vi "DataLog Create Tag Log Directory.vi"(0 "tag log directory":path, 1 "no initial? (false)":bool, 5 "initial number (NaN)":dbl=nan format="%.2f", 7 "initial tag config":T1 {"logging parameters" format="%.2e"; "precision" items=["0", "1", "2", "3", "4", "5", "6", "7", "8", "9", "10", "11", "12", "13", "14", "15", "16", "17"]; "limit delay" format="%.2e"; "deadband" format="%.2e"}, 9 "initial string (\"\")":string, 11 "error in (no error)":errorcluster) -> (4 "dup tag log directory":path, 15 "error out":errorcluster)   [LabVIEW 2012]
doc: "Create a new tag log directory if no such directory exists yet. On creation, a single point with the current time and specified initial value is logged in case of a number tag. In case of a string tag, an undefined string value is logged."
uses:
  typedefs/clusters/t_DataLog Tag Config.ctl
  typedefs/t_DataLog Temporal Types.ctl
  typedefs/t_DataLog Value Types.ctl
  typedefs/t_DataLog Numerical Format.ctl
  typedefs/t_DataLog Logging Algorithms.ctl
  typedefs/clusters/t_DataLog Point.ctl
  glb_DataLog MCVD.vi
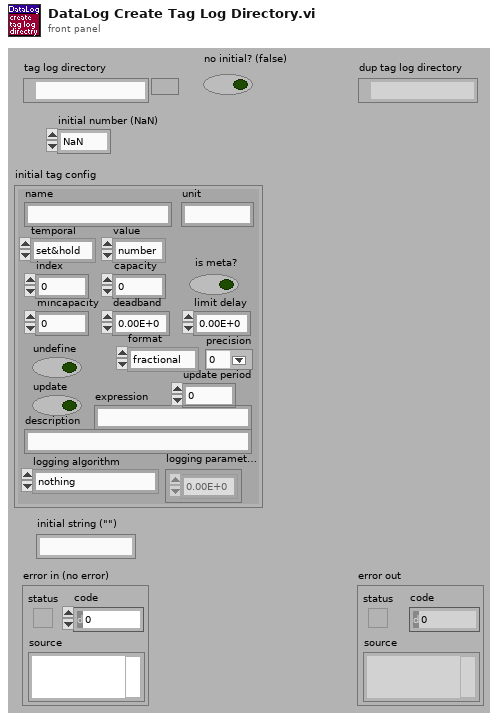
[diagram p1: front panel]
types:
  T1 = typedef "t_DataLog Tag Config.ctl" = cluster{"name":string, "unit":string, "temporal":T2, "value":T3, "index":i32, "capacity":i32, "is meta?":bool, "mincapacity":i32, "deadband":dbl, "limit delay":dbl, "format":T4, "precision":u8, "undefine":bool, "update":bool, "update period":u16, "expression":string, "description":string, "logging algorithm":T5, "logging parameters":dbl[]}
  T2 = typedef "t_DataLog Temporal Types.ctl" = enum16{"set&hold", "sample", "event"}
  T3 = typedef "t_DataLog Value Types.ctl" = enum16{"number", "string"}
  T4 = typedef "t_DataLog Numerical Format.ctl" = enum8{"fractional", "exponential", "engineering"}
  T5 = typedef "t_DataLog Logging Algorithms.ctl" = enum16{"nothing", "changes", "everything", "every Nth", "time threshold", "value threshold + prior", "t or v threshold", "t or v threshold + prior"}
  T6 = enum16{"deny read/write", "deny write-only", "deny none"}
  T7 = typedef "t_DataLog Point.ctl" = cluster{"time":dbl, "value":dbl}
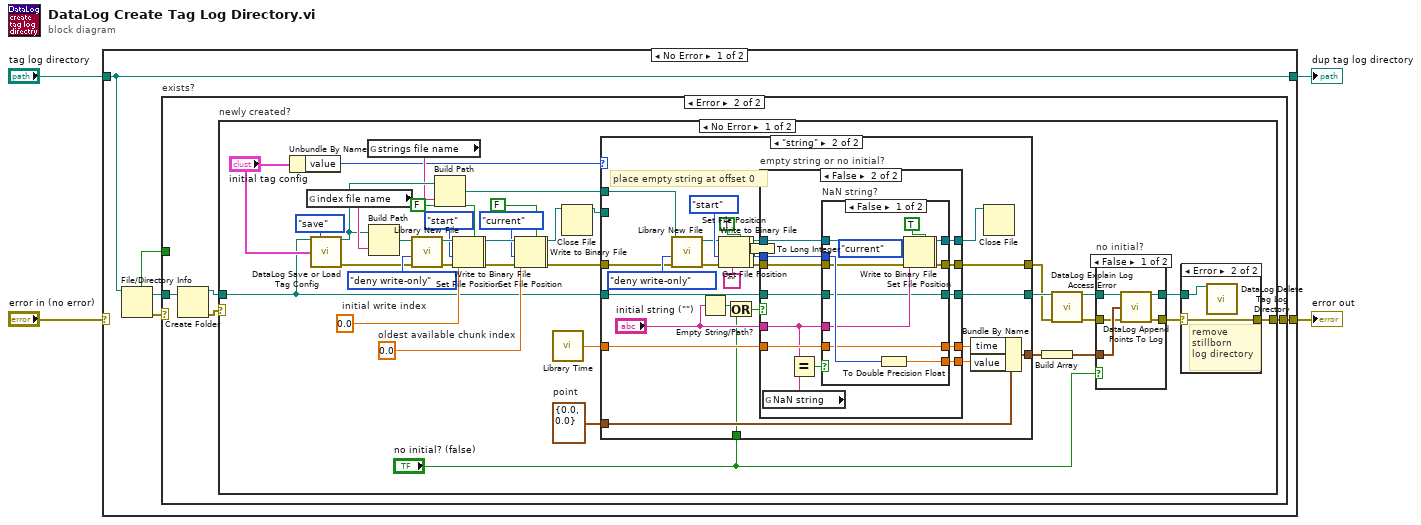
[diagram p0: block diagram]
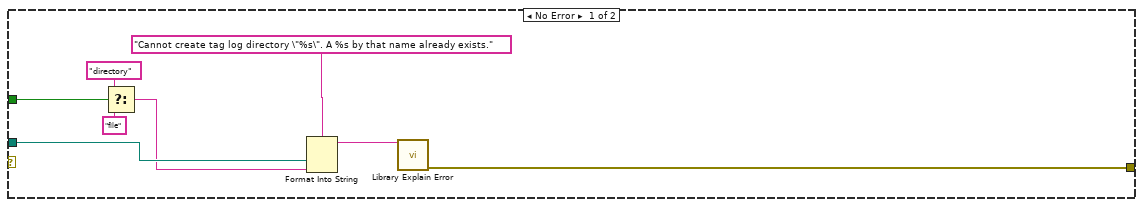
[diagram p2: hidden frame]
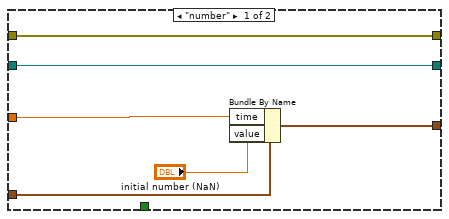
[diagram p4: hidden frame]
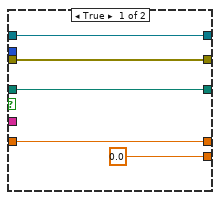
[diagram p5: hidden frame]
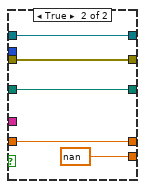
[diagram p6: hidden frame]
diagram:
  n1 = case shown="No Error" "error in (no error)" {
    selector: "error in (no error)" -> [_ w145]
    tunnel: [w9 w145] -> w4
    tunnel: "tag log directory" -> [w7 w144]
    tunnel: [w7 w144] -> w1
    frame No Error {
      n2 = File/Directory Info(path=w7) -> (path out=w8:path, directory=w5:bool, error out=w6:errorcluster)  [unwired: 1 in, 4 out]
      n3 = case "exists?" shown="Error" w6 {
        tunnel: w8 -> [w11 w21]
        tunnel: [w15 w20] -> w9
        tunnel: w5 -> [w14 _]
        frame No Error {
          n4 = Select(t="directory", s=w14, f="file") -> (s? t:f=w10:string)
          n5 = Format Into String(format string="Cannot create tag log directory \"%s\". A %s by that name already exists.", w11, w10) -> (resulting string=w17:string)  [unwired: 2 in, 1 out]
          n6 = call "Library Explain Error.vi"("explanation prefix (none)"=w17) -> ("explained error"=w15:errorcluster)  [unwired: 14 in]
        }
        frame Error {
          n7 = Create Folder(path (use dialog)=w21) -> (created path=w18:path, error out=w19:errorcluster)  [unwired: 2 in, 1 out]
          n8 = case "newly created?" shown="No Error" w19 {
            selector: w19 -> [_ w143]
            tunnel: [w50 w143] -> w20
            tunnel: w18 -> [w34 _]
            frame No Error {
              w35 = T7 {"time"=0.0, "value"=0.0}  # point
              w53 = 0.0  # oldest available chunk index
              w60 = 0.0  # initial write index
              n9 = Unbundle By Name("initial tag config") -> ("value"=w38:T3)
              n10 = global read "glb_DataLog MCVD.vi" "index file name"() -> (w49:string)
              n11 = call "DataLog Save or Load Tag Config.vi"("tag log directory"=w34, "action"=enum16{"save", "load"}."save", "tag config in"="initial tag config") -> ("dup tag log directory"=w44:path, "error out"=w47:errorcluster)  [unwired: 10 in, 1 out]
              n12 = global read "glb_DataLog MCVD.vi" "strings file name"() -> (w43:string)
              n13 = Build Path(base path=w44, name or relative path=w49) -> (appended path=w48:path)
              n14 = call "Library New File.vi"("error in (no error)"=w47, "deny mode (deny none)"=T6."deny write-only" ("deny mode (2)"), "file path"=w48) -> ("error out"=w58:errorcluster, "refnum"=w59:refnum<file>)  [unwired: 7 in]
              n15 = Build Path(base path=w44, name or relative path=w43) -> (appended path=w42:path)
              n16 = Set File Position(refnum=w59, from (0:start)=enum16{"start", "end", "current"}."start" ("pos mode (0:2)"), error in=w58) -> (refnum out=w24:refnum<file>, error out=w23:errorcluster)  [unwired: 1 in]
              n17 = Write to Binary File(file (use dialog)=w24, data=w60, error in=w23, 5:FALSE ("prepend array or string size? (T)")) -> (refnum out=w56:refnum<file>, error out=w54:errorcluster)  [unwired: 2 in, 1 out]
              n18 = Set File Position(refnum=w56, from (0:start)=enum16{"start", "end", "current"}."current" ("pos mode (0:2)"), error in=w54) -> (refnum out=w27:refnum<file>, error out=w26:errorcluster)  [unwired: 1 in]
              n19 = Write to Binary File(file (use dialog)=w27, data=w53, error in=w26, 5:FALSE ("prepend array or string size? (T)")) -> (refnum out=w55:refnum<file>, error out=w45:errorcluster)  [unwired: 2 in, 1 out]
              n20 = call "Library Time.vi"() -> ("time"=w36:dbl)  [unwired: 1 in]
              n21 = Close File(refnum=w55) -> (path=w33:path)  [unwired: 1 in, 1 out]
              n22 = case shown="\"string\"" w38 {
                tunnel: w45 -> [w74 w102]
                tunnel: w42 -> [_ w101]
                tunnel: [w74 w86] -> w29
                tunnel: [w73 w95] -> w37
                tunnel: w36 -> [w72 w85]
                tunnel: w35 -> [w71 w94]
                tunnel: w34 -> [w69 w88]
                tunnel: [w69 w87] -> w32
                tunnel: w33 -> [_ _]
                tunnel: "no initial? (false)" -> [_ w80]
                frame "number" {
                  n23 = Bundle By Name(cluster=w71, "time"=w72, "value"="initial number (NaN)") -> (w73:T7)
                }
                frame "string" {
                  # "place empty string at offset 0"
                  n24 = call "Library New File.vi"("error in (no error)"=w102, "deny mode (deny none)"=T6."deny write-only" ("deny mode (2)"), "file path"=w101) -> ("error out"=w97:errorcluster, "refnum"=w98:refnum<file>)  [unwired: 7 in]
                  n25 = Empty String/Path?(string/path="initial string (\"\")") -> (empty?=w81:bool)
                  n26 = Set File Position(refnum=w98, from (0:start)=enum16{"start", "end", "current"}."start" ("pos mode (0:2)"), error in=w97) -> (refnum out=w79:refnum<file>, error out=w78:errorcluster)  [unwired: 1 in]
                  n27 = Write to Binary File(file (use dialog)=w79, data="", error in=w78, 5:TRUE ("header (F)")) -> (refnum out=w77:refnum<file>, error out=w76:errorcluster)  [unwired: 2 in, 1 out]
                  n28 = Get File Position(4:w76, 7:w77) -> (0:w91:errorcluster, 2:w75:i64, 3:w90:refnum<file>)
                  n29 = Or(x=w81, y=w80) -> (x .or. y?=w82:bool)
                  n30 = To Long Integer(number=w75) -> (32bit integer=w92:i32)
                  n31 = case "empty string or no initial?" shown="False" w82 {
                    tunnel: [0.0 w118] -> w93
                    tunnel: w92 -> [_ w121]
                    tunnel: w91 -> [w108 w120]
                    tunnel: w90 -> [w106 w119]
                    tunnel: [w106 w117] -> w89
                    tunnel: w88 -> [w107 w110]
                    tunnel: [w107 w109] -> w87
                    tunnel: [w108 w116] -> w86
                    tunnel: w85 -> [w104 w114]
                    tunnel: [w104 w115] -> w84
                    tunnel: "initial string (\"\")" -> [_ w113]
                    frame True {
                    }
                    frame False {
                      n32 = global read "glb_DataLog MCVD.vi" "NaN string"() -> (w112:string)
                      n33 = Equal?(x=w113, y=w112) -> (x = y?=w111:bool)
                      n34 = case "NaN string?" shown="False" w111 {
                        tunnel: w121 -> [w132 _]
                        tunnel: w120 -> [w131 w138]
                        tunnel: w119 -> [w130 w139]
                        tunnel: [w129 nan] -> w118
                        tunnel: [w128 w139] -> w117
                        tunnel: [w127 w138] -> w116
                        tunnel: w113 -> [w126 _]
                        tunnel: w114 -> [w125 w137]
                        tunnel: [w125 w137] -> w115
                        tunnel: w110 -> [w124 w135]
                        tunnel: [w124 w135] -> w109
                        frame False {
                          n35 = To Double Precision Float(number=w132) -> (double precision float=w129:dbl)
                          n36 = Set File Position(refnum=w130, from (0:start)=enum16{"start", "end", "current"}."current" ("pos mode (0:2)"), error in=w131) -> (refnum out=w123:refnum<file>, error out=w122:errorcluster)  [unwired: 1 in]
                          n37 = Write to Binary File(file (use dialog)=w123, data=w126, error in=w122, 5:TRUE ("header (F)")) -> (refnum out=w128:refnum<file>, error out=w127:errorcluster)  [unwired: 2 in, 1 out]
                        }
                        frame True {
                        }
                      }
                    }
                  }
                  n38 = Bundle By Name(cluster=w94, "time"=w84, "value"=w93) -> (w95:T7)
                  n39 = Close File(refnum=w89) -> ()  [unwired: 1 in, 2 out]
                }
              }
              n40 = Build Array(w37) -> (w57:T7[])
              n41 = call "DataLog Explain Log Access Error.vi"("tag log directory"=w32, "error in"=w29) -> ("dup tag log directory"=w31:path, "error out"=w30:errorcluster)  [unwired: 12 in]
              n42 = case "no initial?" shown="False" "no initial? (false)" {
                tunnel: w57 -> [w66 _]
                tunnel: [w65 w67] -> w41
                tunnel: [w64 w68] -> w40
                tunnel: w31 -> [w63 w68]
                tunnel: w30 -> [w62 w67]
                frame False {
                  n43 = call "DataLog Append Points To Log.vi"("tag log directory"=w63, "points"=w66, "error in (no error)"=w62) -> ("dup tag log directory"=w64:path, "error out"=w65:errorcluster)  [unwired: 11 in]
                }
                frame True {
                }
              }
              n44 = case shown="Error" w41 {
                selector: w41 -> [w140 w141]
                tunnel: w40 -> [_ w142]
                tunnel: [w140 w141] -> w50
                frame No Error {
                }
                frame Error {
                  # "remove\nstillborn\nlog directory"
                  n45 = call "DataLog Delete Tag Log Directory.vi"("tag log directory"=w142) -> ()  [unwired: 13 in, 2 out]
                }
              }
            }
            frame Error {
            }
          }
        }
      }
    }
    frame Error {
    }
  }
  "error out" <- w4
  "dup tag log directory" <- w1
